vi "DAC Save Results.vi"(8 "error in":errorcluster, 9 "Log Details?":bool, 10 "tdms file":refnum<k34>, 11 "DAC Pressure Scan in":refnum<class "DAC Pressure Scan.lvclass">) -> (0 "error out":errorcluster)   [LabVIEW 2019, in "DAC.lvlib" / "DAC Pressure Scan.lvclass"]
uses:
  DAC Pressure Scan.lvclass
  DAC.lvclass
  C:/Users/krio/Documents/LV_Projects/test-stand/App/DAC/DAC.lvclass
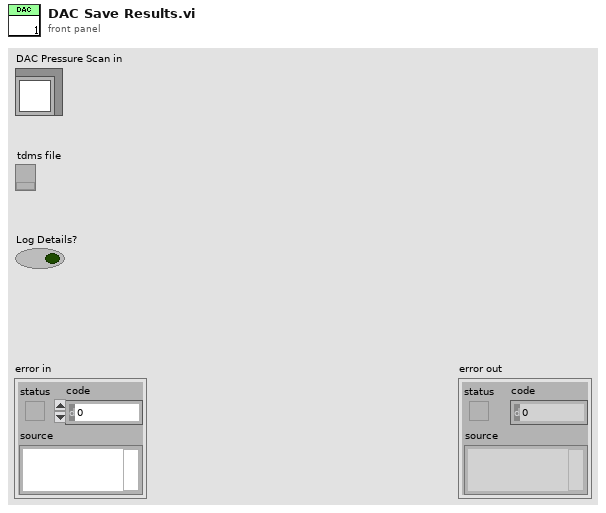
[diagram p1: front panel]
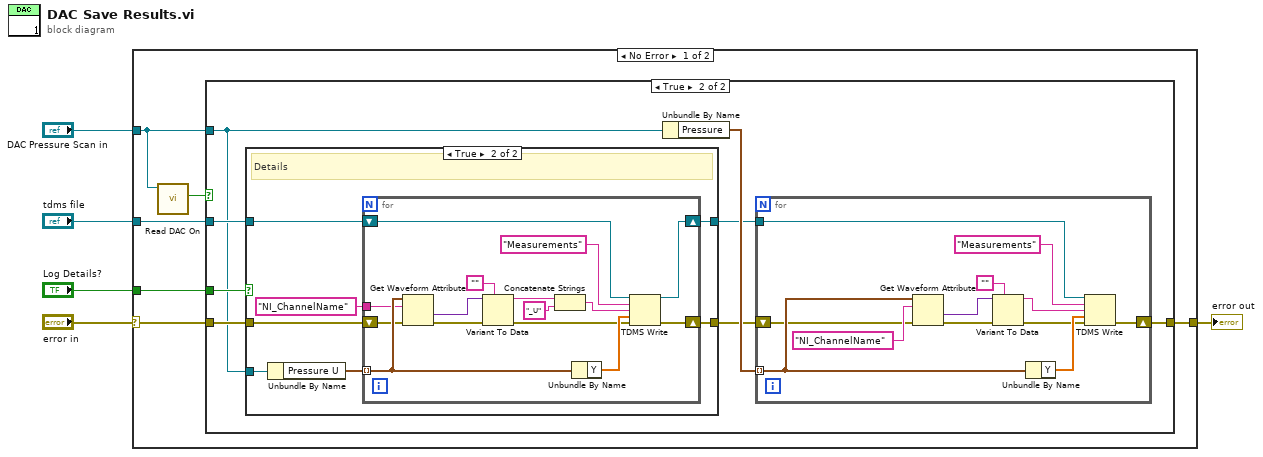
[diagram p0: block diagram]
diagram:
  n1 = case shown="No Error" "error in" {
    selector: "error in" -> [w8 w57]
    tunnel: "DAC Pressure Scan in" -> [w11 _]
    tunnel: "tdms file" -> [w9 _]
    tunnel: [w7 w57] -> w2
    tunnel: "Log Details?" -> [w6 _]
    frame No Error {
      n2 = call "Read DAC On.vi"("DAC in"=w11) -> ("DAC On"=w10:bool)  [unwired: 8 in, 2 out]
      n3 = case shown="True" w10 {
        tunnel: w11 -> [_ w13]
        tunnel: w9 -> [_ w17]
        tunnel: w8 -> [w12 w15]
        tunnel: [w12 w19] -> w7
        tunnel: w6 -> [_ w18]
        frame False {
        }
        frame True {
          n4 = case shown="True" w18 {
            tunnel: w17 -> [w22 w27]
            tunnel: [w22 w23] -> w16
            tunnel: w15 -> [w21 w29]
            tunnel: [w21 w28] -> w14
            tunnel: w13 -> [_ w25]
            frame False {
            }
            frame True {
              # "Details"
              n5 = Unbundle By Name(w25) -> ("Pressure U"=w24:waveform(dbl)[])
              n6 = for {
                tunnel: w24 -> [w39] mode=indexing
                shift-right: [w35] -> w28
                shift-left: w29 -> [w38]
                tunnel: "NI_ChannelName" ("name") -> [w34]
                shift-right: [w30] -> w23
                shift-left: w27 -> [w44]
                n7 = Get Waveform Attribute(4:w38, 6:w34, 7:w39) -> (0:w37:errorcluster, 1:w43:variant)  [unwired: 1 in, 2 out]
                n8 = Variant To Data(error in=w37, type="", Variant=w43) -> (data=w32:string, error out=w36:errorcluster)
                n9 = Concatenate Strings(w32, "_U" ("string")) -> (w33:string)
                n10 = Unbundle By Name(w39) -> ("Y"=w40:dbl[])
                n11 = TDMS Write(0:w44, 5:"Measurements" ("group name in (Untitled)"), 7:w33, 9:w40, 11:w36) -> (4:w30:refnum<k34>, 15:w35:errorcluster)  [unwired: 1 in, 2 out]
              }
            }
          }
          n12 = Unbundle By Name(w13) -> ("Pressure"=w20:waveform(dbl)[])
          n13 = for {
            tunnel: w16 -> [w56]
            tunnel: w20 -> [w49] mode=indexing
            shift-right: [w45] -> w19
            shift-left: w14 -> [w48]
            n14 = Get Waveform Attribute(4:w48, 6:"NI_ChannelName" ("name"), 7:w49) -> (0:w47:errorcluster, 1:w54:variant)  [unwired: 1 in, 2 out]
            n15 = Variant To Data(error in=w47, type="", Variant=w54) -> (data=w50:string, error out=w46:errorcluster)
            n16 = Unbundle By Name(w49) -> ("Y"=w51:dbl[])
            n17 = TDMS Write(0:w56, 5:"Measurements" ("group name in (Untitled)"), 7:w50, 9:w51, 11:w46) -> (15:w45:errorcluster)  [unwired: 1 in, 3 out]
          }
        }
      }
    }
    frame Error {
    }
  }
  "error out" <- w2
